vi "destroyEvent.vi"(8 "error in (no error)":errorcluster, 11 "Event in":refnum<class "Event.lvclass">) -> (0 "error out":errorcluster, 3 "Event out":refnum<class "Event.lvclass">)   [LabVIEW 2009, in "Events.lvlib" / "Event.lvclass"]
uses:
  Event.lvclass
  Event.lvclass/Event.ctl
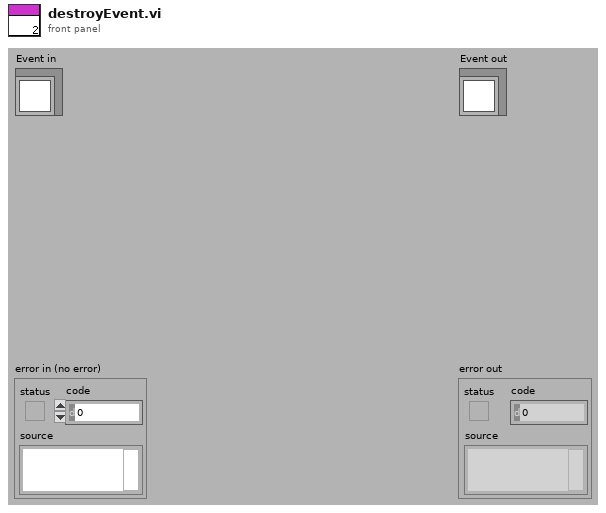
[diagram p1: front panel]
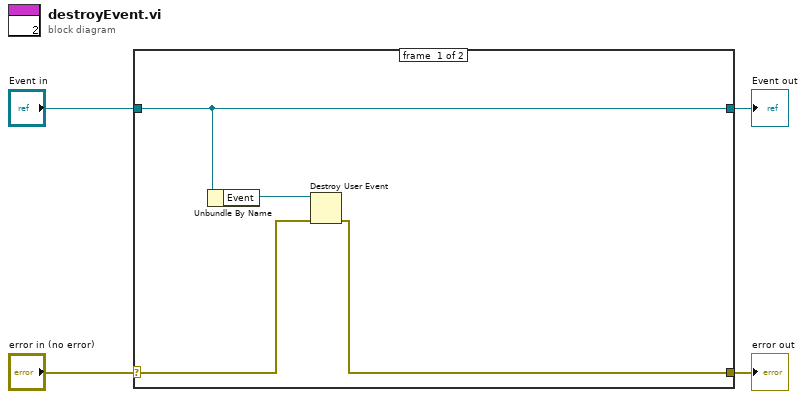
[diagram p0: block diagram]
diagram:
  n1 = case shown="No Error" "error in (no error)" {
    selector: "error in (no error)" -> [w6 w10]
    tunnel: [w5 w10] -> w3
    tunnel: [w8 w9] -> w1
    tunnel: "Event in" -> [w8 w9]
    frame #0 {
      n2 = Unbundle By Name(w8) -> ("Event"=w7:refnum<user-event>)
      n3 = Destroy User Event(user event=w7, error in=w6) -> (error out=w5:errorcluster)
    }
    frame #1 {
    }
  }
  "error out" <- w3
  "Event out" <- w1
